vi "dfd_FXP Filtering with IS.vi"(5 "FXPOPs":T1[](array[typedef]) {"source" items=["Coef a/k"=0, "Coef b/v"=7, "Input"=1, "Output"=2, "Multiplicand"=3, "Product"=4, "Sum"=5, "Delay"=6, "Gain"=8]}, 6 "state in":i64[](array[numeric]), 7 "struct typ":T6=enum."IIR Direct Form II Transposed" caption="structure type", 8 "filtering statistics in":T5(array[cluster]) {"statistics information"."min value" format="%.2f"; "statistics information"."max value" format="%.2f"; "Quantizer Source" items=["Coefficients a/k"=0, "Coefficients b/v"=7, "Input"=1, "Output"=2, "Multiplicand"=3, "Product"=4, "Sum"=5, "Delay"=6]}, 9 "coef a":T7, 10 "coef b":T7, 11 "X":T7) -> (0 "filtering statistics out":T5(array[cluster]) {"statistics information"."min value" format="%.2f"; "statistics information"."max value" format="%.2f"; "Quantizer Source" items=["Coefficients a/k"=0, "Coefficients b/v"=7, "Input"=1, "Output"=2, "Multiplicand"=3, "Product"=4, "Sum"=5, "Delay"=6]}, 3 "filtered X":T7, 4 "state out":i64[](array[numeric]))   [LabVIEW 2017, in "NI_DigFilter_FXP.lvlib"]
uses:
  <vilib>/addons/Digital Filter Design/NI_DigFilter_FXP.lvlib
  <vilib>/addons/Digital Filter Design/_Objects.llb/dfd_DFXP Data Type (vector).ctl
  <vilib>/addons/Digital Filter Design/_Objects.llb/DFD Filter Structure Type Selector.ctl
  <vilib>/addons/Digital Filter Design/_Objects.llb/DFD Quantization Sources.ctl
  <vilib>/addons/Digital Filter Design/_Objects.llb/DFD FXP Statistics Data.ctl
  <vilib>/addons/Digital Filter Design/_Objects.llb/dfd_DFXP Operation Parameter.ctl
  <vilib>/addons/Digital Filter Design/_Objects.llb/dfd_Internal Quantization Srcs.ctl
  <vilib>/addons/Digital Filter Design/NI_DigFilterLicensed.lvlib
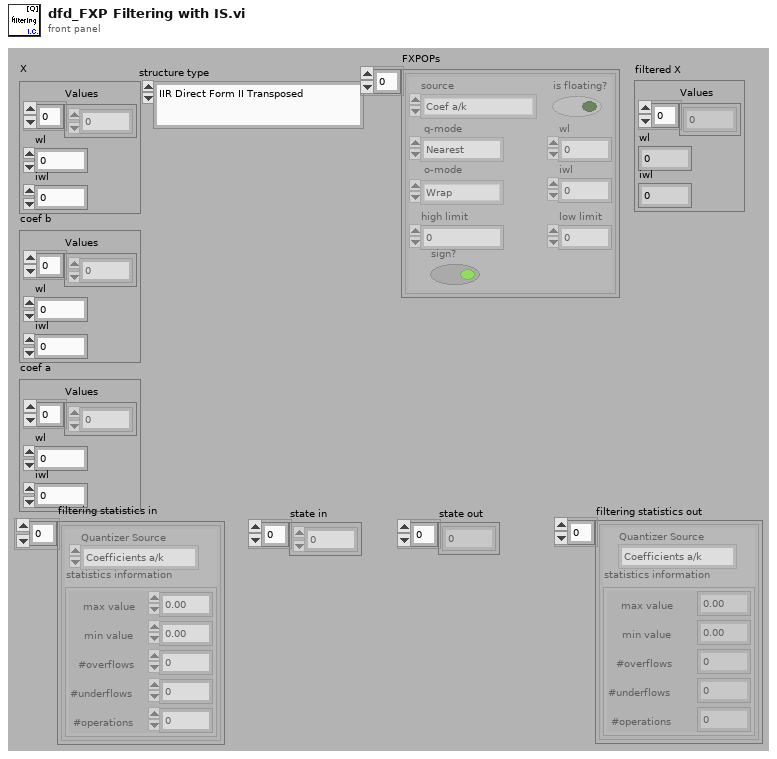
[diagram p1: front panel]
types:
  T1 = typedef "dfd_DFXP Operation Parameter.ctl" = cluster{"source":T2, "is floating?":bool, "o-mode":enum16{"Saturation", "Wrap"}, "q-mode":enum16{"Nearest", "Truncation"}, "wl":i16, "high limit":i64, "low limit":i64, "iwl":i16, "sign?":bool}
  T2 = typedef "NI_DigFilterLicensed.lvlib/dfd_Internal Quantization Srcs.ctl" = u16
  T3 = typedef "NI_DigFilterLicensed.lvlib/DFD Quantization Sources.ctl" = u16
  T4 = typedef "NI_DigFilterLicensed.lvlib/DFD FXP Statistics Data.ctl" = cluster{"max value":ext, "min value":ext, "#overflows":i32, "#underflows":i32, "#operations":i32}
  T5 = cluster{"Quantizer Source":T3, "statistics information":T4}[]
  T6 = typedef "NI_DigFilterLicensed.lvlib/DFD Filter Structure Type Selector.ctl" = enum16{"Undefined", "FIR Direct Form", "FIR Direct Form Transposed", "FIR Symmetric", "FIR Antisymmetric", "IIR Direct Form I", "IIR Direct Form I Transposed", "IIR Direct Form II", "IIR Direct Form II Transposed", "IIR Cascaded Second Order Sections Form I", "IIR Cascaded Second Order Sections Form I Transposed", "IIR Cascaded Second Order Sections Form II", "IIR Cascaded Second Order Sections Form II Transposed", "Lattice Allpass (basic sections)", "Lattice Allpass (one multiplier sections)", "Lattice Allpass (normalized sections)", "Lattice AR (basic sections)", "Lattice AR (one multiplier sections)", "Lattice AR (normalized sections)", "Lattice MA (minimum phase)", "Lattice MA (maximum phase)", "Lattice ARMA (basic sections)", "Lattice ARMA (one multiplier sections)", "Lattice ARMA (normalized sections)"}
  T7 = typedef "dfd_DFXP Data Type (vector).ctl" = cluster{"Values":i64[], "wl":i16, "iwl":i16}
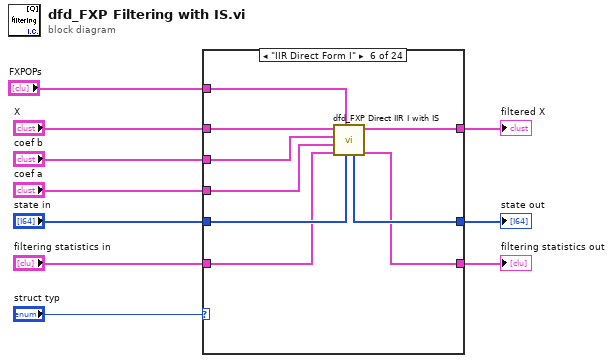
[diagram p0: block diagram]
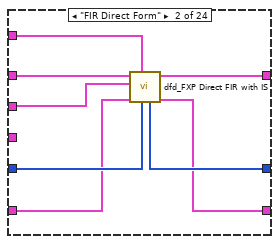
[diagram p3: hidden frame]
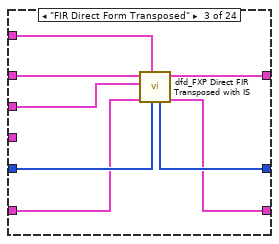
[diagram p4: hidden frame]
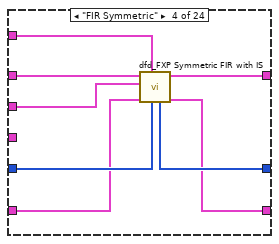
[diagram p5: hidden frame]
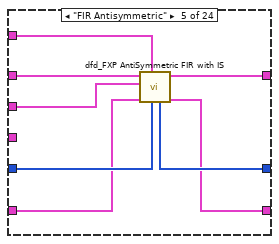
[diagram p6: hidden frame]
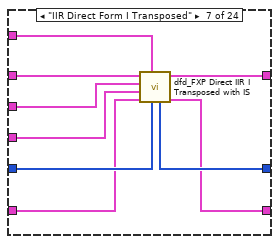
[diagram p7: hidden frame]
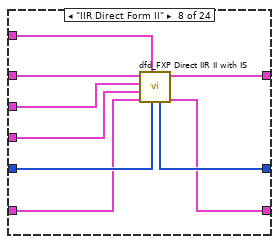
[diagram p8: hidden frame]
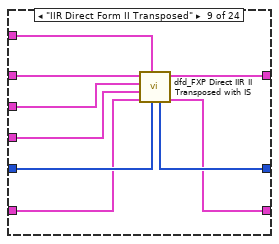
[diagram p9: hidden frame]
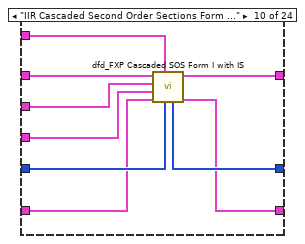
[diagram p10: hidden frame]
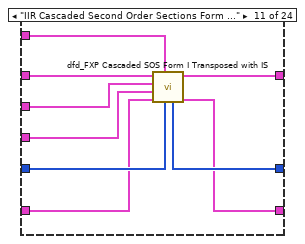
[diagram p11: hidden frame]
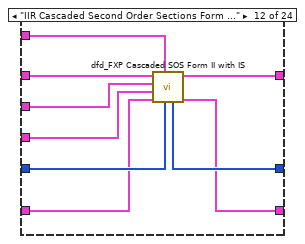
[diagram p12: hidden frame]
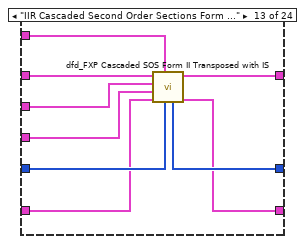
[diagram p13: hidden frame]
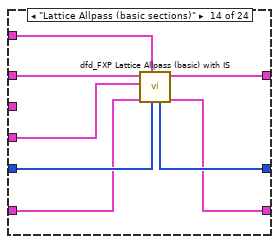
[diagram p14: hidden frame]
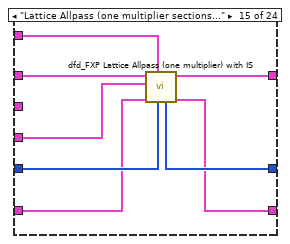
[diagram p15: hidden frame]
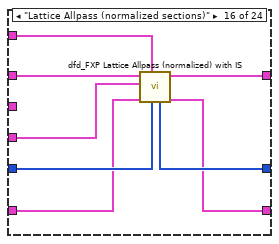
[diagram p16: hidden frame]
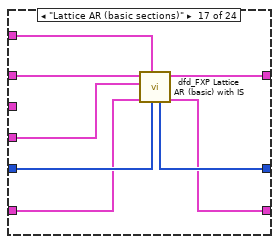
[diagram p17: hidden frame]
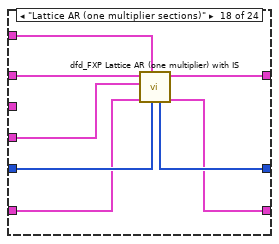
[diagram p18: hidden frame]
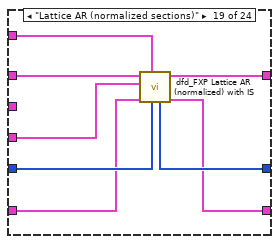
[diagram p19: hidden frame]
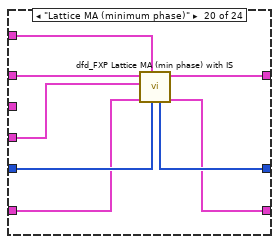
[diagram p20: hidden frame]
diagram:
  n1 = case shown="\"IIR Direct Form I\"" "struct typ" {
    tunnel: "X" -> [_ w20 w28 w36 w44 w53 w62 w71 w80 w89 w98 w107 w116 w124 w132 w140 w148 w156 w164 w172 w180 w189 w198 w207]
    tunnel: "coef b" -> [_ w13 w27 w35 w43 w52 w61 w70 w79 w88 w97 w106 w115 _ _ _ _ _ _ _ _ w188 w197 w206]
    tunnel: "coef a" -> [_ _ _ _ _ w48 w57 w66 w75 w84 w93 w102 w111 w120 w128 w136 w144 w152 w160 w165 w173 w184 w193 w202]
    tunnel: "state in" -> [w12 w19 w26 w34 w42 w51 w60 w69 w78 w87 w96 w105 w114 w123 w131 w139 w147 w155 w163 w171 w179 w187 w196 w205]
    tunnel: [w12 w18 w25 w33 w41 w50 w59 w68 w77 w86 w95 w104 w113 w122 w130 w138 w146 w154 w162 w170 w178 w186 w195 w204] -> w5
    tunnel: [_ w17 w24 w32 w40 w49 w58 w67 w76 w85 w94 w103 w112 w121 w129 w137 w145 w153 w161 w169 w177 w185 w194 w203] -> w4
    tunnel: "FXPOPs" -> [_ w16 w23 w31 w39 w47 w56 w65 w74 w83 w92 w101 w110 w119 w127 w135 w143 w151 w159 w168 w176 w183 w192 w201]
    tunnel: "filtering statistics in" -> [w11 w15 w22 w30 w38 w46 w55 w64 w73 w82 w91 w100 w109 w118 w126 w134 w142 w150 w158 w167 w175 w182 w191 w200]
    tunnel: [w11 w14 w21 w29 w37 w45 w54 w63 w72 w81 w90 w99 w108 w117 w125 w133 w141 w149 w157 w166 w174 w181 w190 w199] -> w2
    frame "Undefined", Default {
    }
    frame "FIR Direct Form" {
      n2 = call <vilib>:"dfd_FXP Direct FIR with IS.vi"("state in"=w19, "FXPOPs"=w16, "filtering statistics in"=w15, "coef b"=w13, "X"=w20) -> ("filtering statistics out"=w14:T5, "filtered X"=w17:T7, "state out"=w18:i64[])  [unwired: 4 out]
    }
    frame "FIR Direct Form Transposed" {
      n3 = call <vilib>:"dfd_FXP Direct FIR Transposed with IS.vi"("state in"=w26, "FXPOPs"=w23, "filtering statistics in"=w22, "coef b"=w27, "X"=w28) -> ("filtering statistics out"=w21:T5, "filtered X"=w24:T7, "state out"=w25:i64[])  [unwired: 4 out]
    }
    frame "FIR Symmetric" {
      n4 = call <vilib>:"dfd_FXP Symmetric FIR with IS.vi"("state in"=w34, "FXPOPs"=w31, "filtering statistics in"=w30, "coef b"=w35, "X"=w36) -> ("filtering statistics out"=w29:T5, "filtered X"=w32:T7, "state out"=w33:i64[])  [unwired: 4 out]
    }
    frame "FIR Antisymmetric" {
      n5 = call <vilib>:"dfd_FXP AntiSymmetric FIR with IS.vi"("state in"=w42, "FXPOPs"=w39, "filtering statistics in"=w38, "coef b"=w43, "X"=w44) -> ("filtering statistics out"=w37:T5, "filtered X"=w40:T7, "state out"=w41:i64[])  [unwired: 4 out]
    }
    frame "IIR Direct Form I" {
      n6 = call <vilib>:"dfd_FXP Direct IIR I with IS.vi"("state in"=w51, "FXPOPs"=w47, "filtering statistics in"=w46, "coef a"=w48, "coef b"=w52, "X"=w53) -> ("filtering statistics out"=w45:T5, "filtered X"=w49:T7, "state out"=w50:i64[])  [unwired: 3 out]
    }
    frame "IIR Direct Form I Transposed" {
      n7 = call <vilib>:"dfd_FXP Direct IIR I Transposed with IS.vi"("state in"=w60, "quantizers"=w56, "filtering statistics in"=w55, "coef a"=w57, "coef b"=w61, "X"=w62) -> ("filtering statistics out"=w54:T5, "filtered X"=w58:T7, "state out"=w59:i64[])  [unwired: 3 out]
    }
    frame "IIR Direct Form II" {
      n8 = call <vilib>:"dfd_FXP Direct IIR II with IS.vi"("state in"=w69, "quantizers"=w65, "filtering statistics in"=w64, "coef a"=w66, "coef b"=w70, "X"=w71) -> ("filtering statistics out"=w63:T5, "filtered X"=w67:T7, "state out"=w68:i64[])  [unwired: 3 out]
    }
    frame "IIR Direct Form II Transposed" {
      n9 = call <vilib>:"dfd_FXP Direct IIR II Transposed with IS.vi"("state in"=w78, "quantizers"=w74, "filtering statistics in"=w73, "coef a"=w75, "coef b"=w79, "X"=w80) -> ("filtering statistics out"=w72:T5, "filtered X"=w76:T7, "state out"=w77:i64[])  [unwired: 3 out]
    }
    frame "IIR Cascaded Second Order Sections Form I" {
      n10 = call <vilib>:"dfd_FXP Cascaded SOS Form I with IS.vi"("state in"=w87, "quantizers"=w83, "filtering statistics in"=w82, "coef a"=w84, "coef b"=w88, "X"=w89) -> ("filtering statistics out"=w81:T5, "filtered X"=w85:T7, "state out"=w86:i64[])  [unwired: 3 out]
    }
    frame "IIR Cascaded Second Order Sections Form I Transposed" {
      n11 = call <vilib>:"dfd_FXP Cascaded SOS Form I Transposed with IS.vi"("state in"=w96, "quantizers"=w92, "filtering statistics in"=w91, "coef a"=w93, "coef b"=w97, "X"=w98) -> ("filtering statistics out"=w90:T5, "filtered X"=w94:T7, "state out"=w95:i64[])  [unwired: 3 out]
    }
    frame "IIR Cascaded Second Order Sections Form II" {
      n12 = call <vilib>:"dfd_FXP Cascaded SOS Form II with IS.vi"("state in"=w105, "quantizers"=w101, "filtering statistics in"=w100, "coef a"=w102, "coef b"=w106, "X"=w107) -> ("filtering statistics out"=w99:T5, "filtered X"=w103:T7, "state out"=w104:i64[])  [unwired: 3 out]
    }
    frame "IIR Cascaded Second Order Sections Form II Transposed" {
      n13 = call <vilib>:"dfd_FXP Cascaded SOS Form II Transposed with IS.vi"("state in"=w114, "FXPOPs"=w110, "filtering statistics in"=w109, "coef a"=w111, "coef b"=w115, "X"=w116) -> ("filtering statistics out"=w108:T5, "filtered X"=w112:T7, "state out"=w113:i64[])  [unwired: 3 out]
    }
    frame "Lattice Allpass (basic sections)" {
      n14 = call <vilib>:"dfd_FXP Lattice Allpass (basic) with IS.vi"("state in"=w123, "FXPOPs"=w119, "filtering statistics in"=w118, "coef k"=w120, "X"=w124) -> ("filtering statistics out"=w117:T5, "filtered X"=w121:T7, "state out"=w122:i64[])  [unwired: 4 out]
    }
    frame "Lattice Allpass (one multiplier sections)" {
      n15 = call <vilib>:"dfd_FXP Lattice Allpass (one multiplier) with IS.vi"("state in"=w131, "FXPOPs"=w127, "filtering statistics in"=w126, "coef k"=w128, "X"=w132) -> ("filtering statistics out"=w125:T5, "filtered X"=w129:T7, "state out"=w130:i64[])  [unwired: 4 out]
    }
    frame "Lattice Allpass (normalized sections)" {
      n16 = call <vilib>:"dfd_FXP Lattice Allpass (normalized) with IS.vi"("state in"=w139, "FXPOPs"=w135, "filtering statistics in"=w134, "coef k & ^k"=w136, "X"=w140) -> ("filtering statistics out"=w133:T5, "filtered X"=w137:T7, "state out"=w138:i64[])  [unwired: 4 out]
    }
    frame "Lattice AR (basic sections)" {
      n17 = call <vilib>:"dfd_FXP Lattice AR (basic) with IS.vi"("state in"=w147, "FXPOPs"=w143, "filtering statistics in"=w142, "coef k"=w144, "X"=w148) -> ("filtering statistics out"=w141:T5, "filtered X"=w145:T7, "state out"=w146:i64[])  [unwired: 4 out]
    }
    frame "Lattice AR (one multiplier sections)" {
      n18 = call <vilib>:"dfd_FXP Lattice AR (one multiplier) with IS.vi"("state in"=w155, "FXPOPs"=w151, "filtering statistics in"=w150, "coef k"=w152, "X"=w156) -> ("filtering statistics out"=w149:T5, "filtered X"=w153:T7, "state out"=w154:i64[])  [unwired: 4 out]
    }
    frame "Lattice AR (normalized sections)" {
      n19 = call <vilib>:"dfd_FXP Lattice AR (normalized) with IS.vi"("state in"=w163, "FXPOPs"=w159, "filtering statistics in"=w158, "coef k & ^k"=w160, "X"=w164) -> ("filtering statistics out"=w157:T5, "filtered X"=w161:T7, "state out"=w162:i64[])  [unwired: 4 out]
    }
    frame "Lattice MA (minimum phase)" {
      n20 = call <vilib>:"dfd_FXP Lattice MA (min phase) with IS.vi"("state in"=w171, "FXPOPs"=w168, "filtering statistics in"=w167, "coef k"=w165, "X"=w172) -> ("filtering statistics out"=w166:T5, "filtered X"=w169:T7, "state out"=w170:i64[])  [unwired: 4 out]
    }
    frame "Lattice MA (maximum phase)" {
      n21 = call <vilib>:"dfd_FXP Lattice MA (max phase) with IS.vi"("state in"=w179, "FXPOPs"=w176, "filtering statistics in"=w175, "coef k"=w173, "X"=w180) -> ("filtering statistics out"=w174:T5, "filtered X"=w177:T7, "state out"=w178:i64[])  [unwired: 4 out]
    }
    frame "Lattice ARMA (basic sections)" {
      n22 = call <vilib>:"dfd_FXP Lattice ARMA (basic) with IS.vi"("state in"=w187, "FXPOPs"=w183, "filtering statistics in"=w182, "coef v"=w188, "coef k"=w184, "X"=w189) -> ("filtering statistics out"=w181:T5, "filtered X"=w185:T7, "state out"=w186:i64[])  [unwired: 3 out]
    }
    frame "Lattice ARMA (one multiplier sections)" {
      n23 = call <vilib>:"dfd_FXP Lattice ARMA (one multiplier) with IS.vi"("state in"=w196, "FXPOPs"=w192, "filtering statistics in"=w191, "coef v"=w197, "coef k"=w193, "X"=w198) -> ("filtering statistics out"=w190:T5, "filtered X"=w194:T7, "state out"=w195:i64[])  [unwired: 3 out]
    }
    frame "Lattice ARMA (normalized sections)" {
      n24 = call <vilib>:"dfd_FXP Lattice ARMA (normalized) with IS.vi"("state in"=w205, "FXPOPs"=w201, "filtering statistics in"=w200, "coef v"=w206, "coef k & ^k"=w202, "X"=w207) -> ("filtering statistics out"=w199:T5, "filtered X"=w203:T7, "state out"=w204:i64[])  [unwired: 3 out]
    }
  }
  "state out" <- w5
  "filtered X" <- w4
  "filtering statistics out" <- w2
